vi "Parse Monitor Record (Multiple).vi"(9 "record count":i32, 10 "header size bytes (32)":i32=32, 11 "Record In":u8[](array[numeric])) -> (0 "HeaderInfo":T3[](array[typedef]) {"FHW0"."MacID" format="%03b"}, 1 "BECW":T7[](array[typedef]), 2 "Payloads":T1[](array[typedef]), 3 "Record Out":u8[](array[numeric]))   [LabVIEW 2020]
uses:
  <instrlib>/AIM GmbH/_AIM 664/AIM664LV.lvlib
  <instrlib>/AIM GmbH/_AIM 664/_controls/monitor_fhw0_type.ctl
  <instrlib>/AIM GmbH/_AIM 664/_controls/monitor_fhw1_type.ctl
  <instrlib>/AIM GmbH/_AIM 664/_controls/monitor_entrySize_type.ctl
  <instrlib>/AIM GmbH/_AIM 664/_controls/monitor_fhInfol_type.ctl
  Frame.ctl
  <instrlib>/AIM GmbH/_AIM 664/_controls/monitor_becw_type.ctl
panel:
  in  "byte order (0:big-endian, network order)":T2(ring)=enum."native, host order"
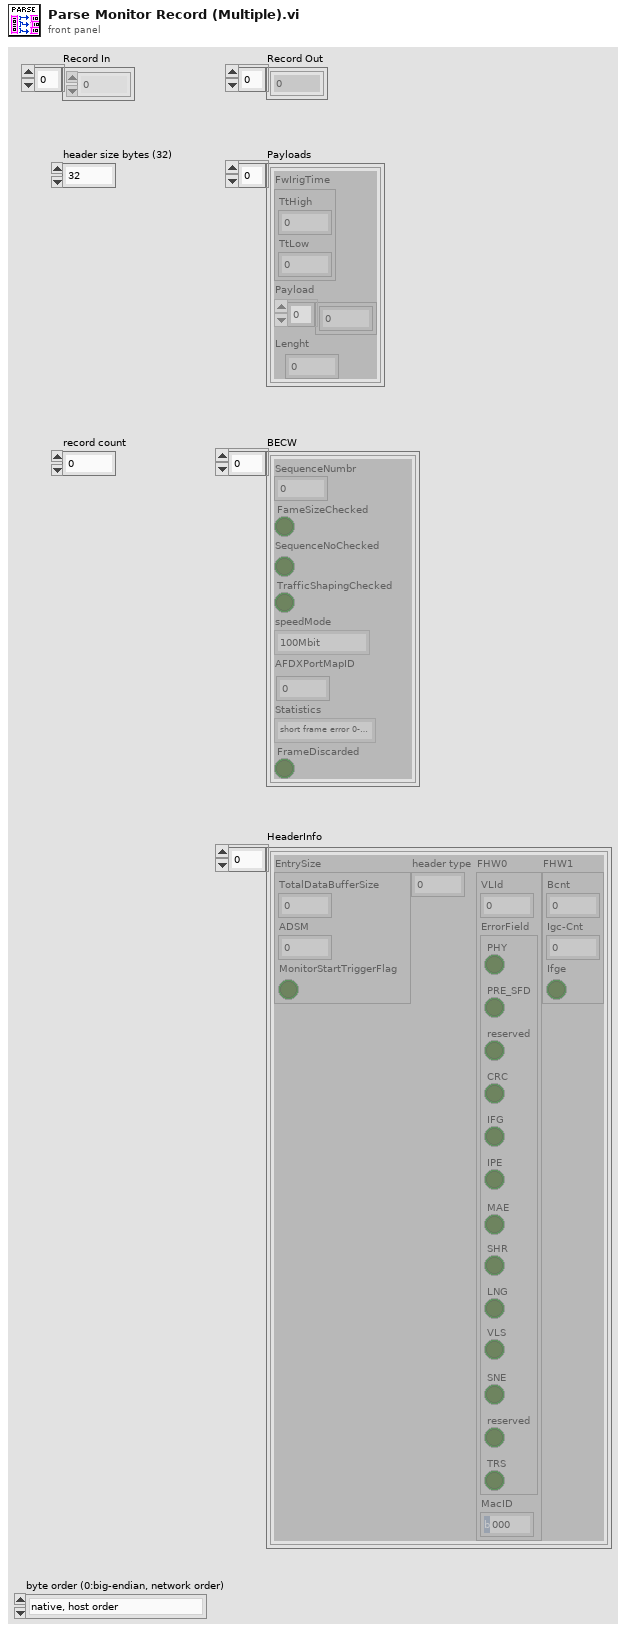
[diagram p1: front panel]
types:
  T1 = typedef "Frame.ctl" = cluster{"FwIrigTime":cluster{"TtHigh":u32, "TtLow":u32}, "Payload":u8[], "Lenght":u32}
  T2 = enum16{"big-endian, network order", "native, host order", "little-endian"}
  T3 = typedef "AIM664LV.lvlib/monitor_fhInfol_type.ctl" = cluster{"EntrySize":T4, "header type":u32, "FHW0":T5, "FHW1":T6}
  T4 = typedef "AIM664LV.lvlib/monitor_entrySize_type.ctl" = cluster{"TotalDataBufferSize":u16, "ADSM":u16, "MonitorStartTriggerFlag":bool}
  T5 = typedef "AIM664LV.lvlib/monitor_fhw0_type.ctl" = cluster{"VLId":u16, "ErrorField":cluster{"PHY":bool, "PRE_SFD":bool, "reserved":bool, "CRC":bool, "IFG":bool, "IPE":bool, "MAE":bool, "SHR":bool, "LNG":bool, "VLS":bool, "SNE":bool, "reserved":bool, "TRS":bool}, "MacID":u8}
  T6 = typedef "AIM664LV.lvlib/monitor_fhw1_type.ctl" = cluster{"Bcnt":u16, "Igc-Cnt":u16, "Ifge":bool}
  T7 = typedef "AIM664LV.lvlib/monitor_becw_type.ctl" = cluster{"SequenceNumbr":u8, "FameSizeChecked":bool, "SequenceNoChecked":bool, "TrafficShapingChecked":bool, "speedMode":enum16{"100Mbit", "10Mbit", "1Gbit"}, "AFDXPortMapID":u8, "Statistics":enum16{"short frame error 0-63Bytes", "64-127 Bytes", "128-255 Bytes", "256-511 Bytes", "512-1023 Bytes", "1024-1518 Bytes", ">1518 Bytes"}, "FrameDiscarded":bool}
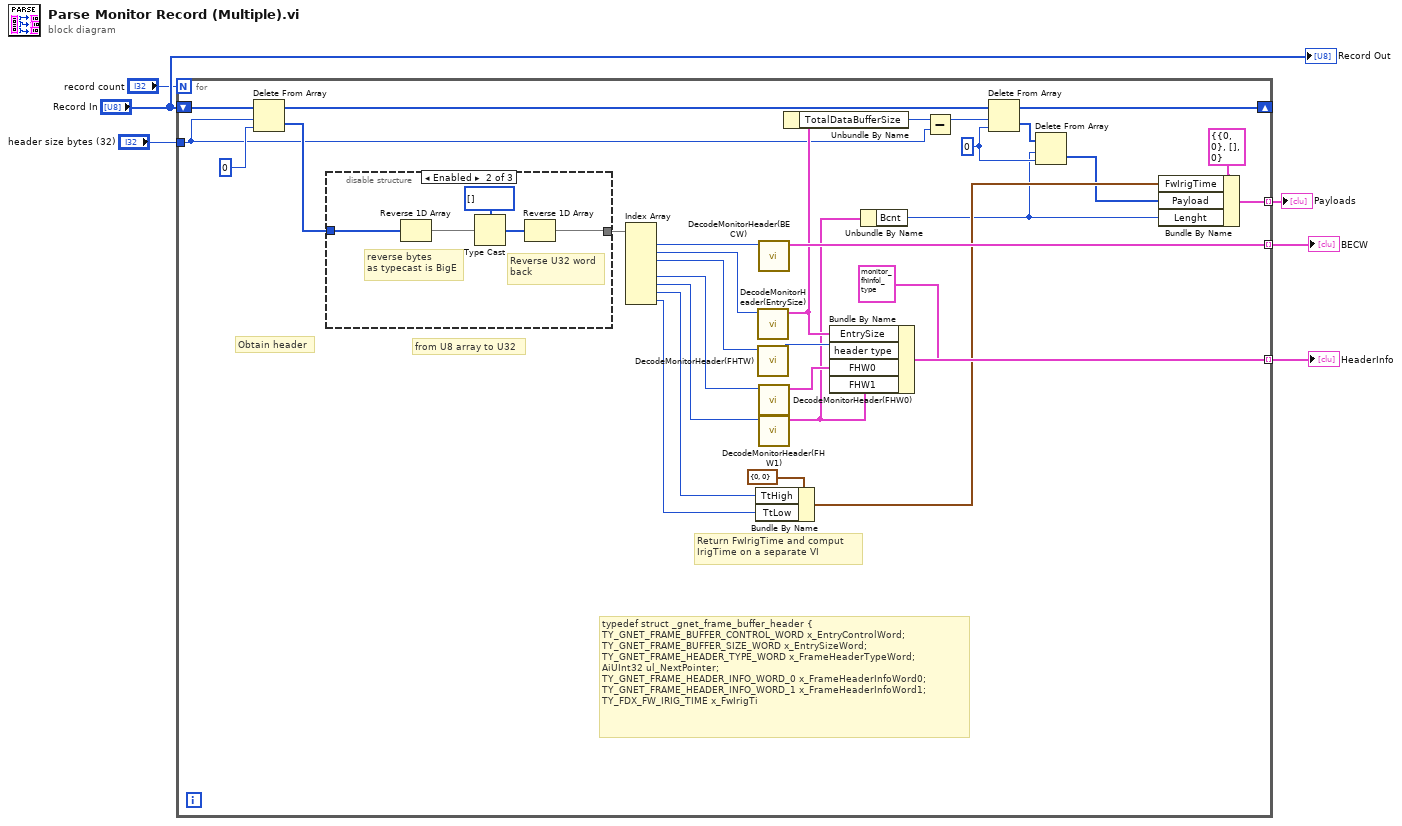
[diagram p0: block diagram]
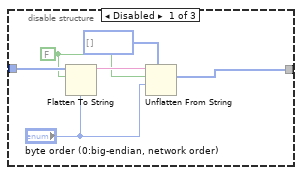
[diagram p2: hidden frame]
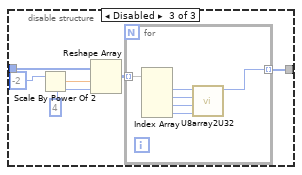
[diagram p3: hidden frame]
diagram:
  n1 = for {
    N: "record count" -> [_]
    tunnel: [w37] -> w6 mode=indexing
    tunnel: [w36] -> w5 mode=indexing
    tunnel: "header size bytes (32)" -> [w7]
    shift-right: [w16] -> _
    shift-left: "Record In" -> [w19]
    tunnel: [w17] -> w2 mode=indexing
    w12 = 0
    # "Return FwIrigTime and comput\nIrigTime on a separate VI"
    # "typedef struct _gnet_frame_buffer_header {\nTY_GNET_FRAME_BUFFER_CONTROL_WORD x_EntryControlWord;\nTY_GNET_FRAME_BUFFER_SIZE_WORD x_EntrySizeWord;\nTY_GNET_FRAME_HEADER_TYPE_WORD x_FrameHeaderTypeWord;\nAiUInt32 ul_NextPointer;\nTY_GNET_FRAME_HEADER_INFO_WORD_0 x_FrameHeaderInfoWord0;\nTY_GNET_FRAME_HEADER_INFO_WORD_1 x_FrameHeaderInfoWord1;\nTY_FDX_FW_IRIG_TIME x_FwIrigTi"
    # "from U8 array to U32"
    # "Obtain header"
    n2 = Delete From Array(array=w19, length=w7, index=0) -> (deleted portion=w33:u8[], array with subset deleted=w18:u8[])
    n3 = disable-structure shown="Enabled" {
      disable-tunnel: [w40 w44 w52] -> w35
      disable-tunnel: w33 -> [w43 w48 w54]
      frame Disabled {
        w39 = FALSE ("prepend array or string size? (T)")
        n4 = Flatten To String(anything=w43, prepend array or string size? (T)=w39, byte order (0:big-endian, network order)="byte order (0:big-endian, network order)") -> (data string=w41:string)  [unwired: 1 in, 2 out]
        n5 = Unflatten From String(type=u32[] [] ("index"), binary string=w41, data includes array or string size? (T)=w39, byte order (0:big-endian, network order)="byte order (0:big-endian, network order)") -> (value=w40:u32[])  [unwired: 1 in, 2 out]
      }
      frame Enabled {
        # "Reverse U32 word\nback"
        # "reverse bytes\nas typecast is BigE"
        n6 = Reverse 1D Array(array=w48) -> (reversed array=w47:u8[])
        n7 = Type Cast(type=u32[] [] ("index"), x=w47) -> (*(type *) &x=w45:u32[])
        n8 = Reverse 1D Array(array=w45) -> (reversed array=w44:u32[])
      }
      frame Disabled {
        n9 = Scale By Power Of 2(n=i16 -2) -> (x*2^n=w49:ext)  [unwired: 1 in]
        n10 = Reshape Array(w54, w49, i16 4 ("n")) -> (w53:u8[][])
        n11 = for {
          tunnel: w53 -> [w60] mode=indexing
          tunnel: [w55] -> w52 mode=indexing
          n12 = Index Array(array=w60) -> (element #1=w59:u8, element #2=w58:u8, element #3=w57:u8, element #4=w56:u8)  [unwired: 4 in]
          n13 = call "U8array2U32.vi"("hi 2"=w56, "lo 2"=w57, "hi"=w58, "lo"=w59) -> ("(hi.lo)"=w55:u32)  [unwired: 7 in]
        }
      }
    }
    n14 = Index Array(array=w35) -> (element #1=w27:u32, element #2=w23:u32, element #3=w24:u32, element #5=w28:u32, element #6=w29:u32, element #7=w31:u32, element #8=w30:u32)  [unwired: 8 in, 1 out]
    n15 = Bundle By Name(cluster=cluster{"TtHigh":u32, "TtLow":u32} {"TtHigh"=0, "TtLow"=0} ("FwIrigTime"), "TtHigh"=w31, "TtLow"=w30) -> (w20:cluster{"TtHigh":u32, "TtLow":u32})
    n16 = call <instrlib>:"DecodeMonitorHeader(EntrySize).vi"("EntrySizeWord"=w23) -> ("EntrySize"=w15:T4)  [unwired: 10 in]
    n17 = call <instrlib>:"DecodeMonitorHeader(FHTW).vi"("fhtw"=w24) -> ("header type"=w25:u32)  [unwired: 10 in]
    n18 = call <instrlib>:"DecodeMonitorHeader(BECW).vi"("becw"=w27) -> ("BECW"=w37:T7)  [unwired: 10 in]
    n19 = call <instrlib>:"DecodeMonitorHeader(FHW0).vi"("fhw0"=w28) -> ("FHW0"=w26:T5)  [unwired: 10 in]
    n20 = call <instrlib>:"DecodeMonitorHeader(FHW1).vi"("fhw1"=w29) -> ("FHW1"=w11:T6)  [unwired: 10 in]
    n21 = Unbundle By Name(w15) -> ("TotalDataBufferSize"=w14:u16)
    n22 = Bundle By Name(cluster=T3 {"EntrySize"={"TotalDataBufferSize"=0, "ADSM"=0, "MonitorStartTriggerFlag"=FALSE}, "header type"=0, "FHW0"={"VLId"=0, "ErrorField"={"PHY"=FALSE, "PRE_SFD"=FALSE, "reserved"=FALSE, "CRC"=FALSE, "IFG"=FALSE, "IPE"=FALSE, "MAE"=FALSE, "SHR"=FALSE, "LNG"=FALSE, "VLS"=FALSE, "SNE"=FALSE, "reserved"=FALSE, "TRS"=FALSE}, "MacID"=0}, "FHW1"={"Bcnt"=0, "Igc-Cnt"=0, "Ifge"=FALSE}} ("FrameHeaderInfo"), "EntrySize"=w15, "header type"=w25, "FHW0"=w26, "FHW1"=w11) -> (w36:T3)
    n23 = Unbundle By Name(w11) -> ("Bcnt"=w10:u16)
    n24 = Subtract(x=w14, y=w7) -> (x-y=w8:i32)
    n25 = Delete From Array(array=w18, length=w8, index=w12) -> (deleted portion=w13:u8[], array with subset deleted=w16:u8[])
    n26 = Delete From Array(array=w13, length=w10, index=w12) -> (deleted portion=w9:u8[])  [unwired: 1 out]
    n27 = Bundle By Name(cluster=T1 {"FwIrigTime"={"TtHigh"=0, "TtLow"=0}, "Payload"=[], "Lenght"=0} ("Frame"), "FwIrigTime"=w20, "Payload"=w9, "Lenght"=w10) -> (w17:T1)
  }
  "BECW" <- w6
  "HeaderInfo" <- w5
  "Payloads" <- w2
  "Record Out" <- "Record In"
